vi "ActDriveStraightCommon.vi"(10 "FirstTime":bool, 11 "Dist (ft)":dbl) -> (3 "Error":dbl)   [LabVIEW 2023]
uses:
  <vilib>/Rock Robotics/Network Tables/NT Write Numeric Array.vi
  <vilib>/Rock Robotics/Network Tables/NT Write Boolean.vi
  <vilib>/Rock Robotics/Network Tables/NT Write Number.vi
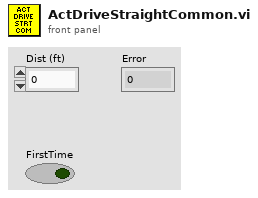
[diagram p1: front panel]
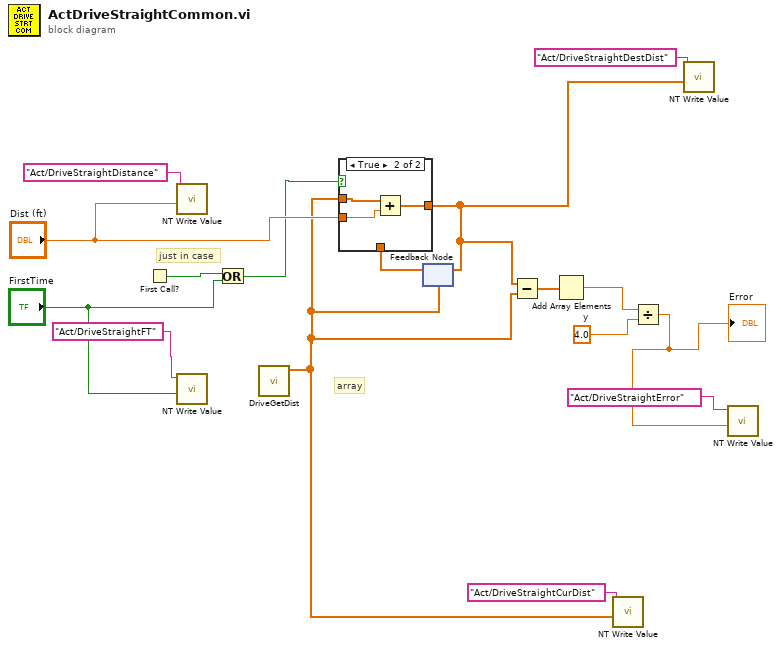
[diagram p0: block diagram]
diagram:
  w10 = 4.0  # y
  # "just in case"
  # "array"
  n1 = First Call?() -> (First Call?: T/F=w3:bool)
  n2 = call-poly <vilib>:"NT Write Value.vi"("value"="Dist (ft)", "name"="Act/DriveStraightDistance") -> ()  [unwired: 9 in, 1 out]
  n3 = call-poly <vilib>:"NT Write Value.vi"("value"="FirstTime", "name"="Act/DriveStraightFT") -> ()  [unwired: 9 in, 1 out]
  n4 = Or(x=w3, y="FirstTime") -> (x .or. y?=w1:bool)
  n5 = call "DriveGetDist.vi"() -> ("ModuleTravelPosition"=w4:dbl[])  [unwired: 11 in]
  n6 = feedback #1(w4) -> (w15:dbl[])
  n7 = case shown="True" w1 {
    tunnel: "Dist (ft)" -> [_ w19]
    tunnel: w4 -> [_ w20]
    tunnel: [w17 w18] -> w6
    tunnel: w15 -> [w17 _]
    frame False {
    }
    frame True {
      n8 = Add(x=w20, y=w19) -> (x+y=w18:dbl[])
    }
  }
  n9 = feedback-in #1(w6) -> ()
  n10 = Subtract(x=w6, y=w4) -> (x-y=w16:dbl[])
  n11 = Add Array Elements(numeric array=w16) -> (sum=w9:dbl)
  n12 = call-poly <vilib>:"NT Write Value.vi"("value"=w4, "name"="Act/DriveStraightCurDist") -> ()  [unwired: 9 in, 1 out]
  n13 = Divide(x=w9, y=w10) -> (x/y=w8:dbl)
  "Error" <- w8
  n14 = call-poly <vilib>:"NT Write Value.vi"("value"=w6, "name"="Act/DriveStraightDestDist") -> ()  [unwired: 9 in, 1 out]
  n15 = call-poly <vilib>:"NT Write Value.vi"("value"=w8, "name"="Act/DriveStraightError") -> ()  [unwired: 9 in, 1 out]
